vi "Get Static Boolean.vi"(8 "error in (no error)":errorcluster, 9 "Tag":string, 10 "Value Type":refnum<class "Abs_Boolean.lvclass">, 11 "Var Bus in":refnum<class "Multi_Bus.lvclass">) -> (0 "error out":errorcluster, 2 "Value Out":refnum<class "Abs_Boolean.lvclass">, 3 "Var Bus out":refnum<class "Multi_Bus.lvclass">)   [LabVIEW 2021, in "Multi_Bus.lvclass"]
uses:
  Multi_Bus.lvclass
  Multi_Bus.lvclass/Multi_Bus.ctl
  <vilib>/TSA/Abstract Data Classes/Abs_Types/Boolean/Abs_Boolean.lvclass
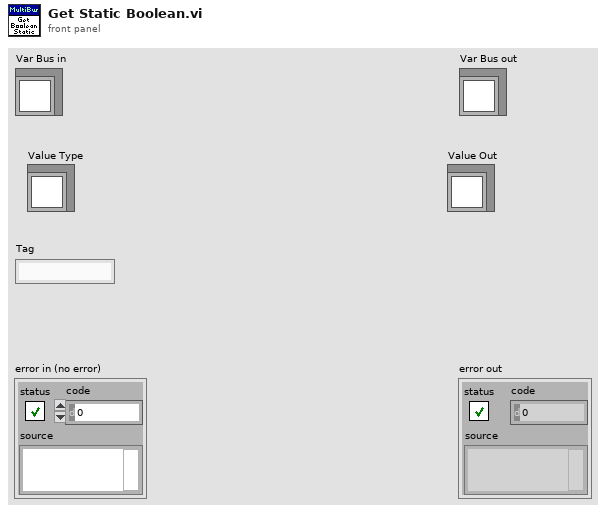
[diagram p1: front panel]
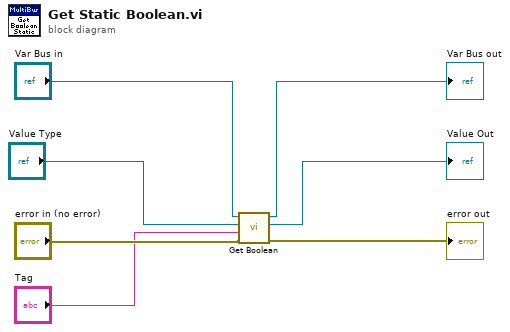
[diagram p0: block diagram]
diagram:
  n1 = call-dynamic "Get Boolean.vi"("error in (no error)"="error in (no error)", "Tag"="Tag", "Value Type"="Value Type", "Var Bus in"="Var Bus in") -> ("error out"=→"error out":errorcluster, "Value Out"=→"Value Out":refnum<class "Abs_Boolean.lvclass">, "Var Bus out"=→"Var Bus out":refnum<class "Multi_Bus.lvclass">)  [unwired: 5 in]
